vi "E5_ExDiag.vi"() -> ()   [LabVIEW 2025]
panel:
  out "subarray":dbl[](array[numeric])
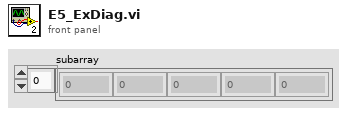
[diagram p1: front panel]
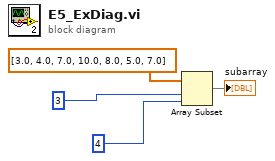
[diagram p0: block diagram]
diagram:
  n1 = Array Subset "Array Subset"(array=dbl[] [3.0, 4.0, 7.0, 10.0, 8.0, 5.0, 7.0], index=3, length=4) -> (→"subarray":dbl[])
